vi "close.vi"(8 "error in (no error)":errorcluster, 11 "K2602 in":refnum<class "K2602.lvclass">) -> (0 "error out":errorcluster)   [LabVIEW 2009, in "Hardware.lvlib" / "Channels.lvlib" / "K2602.lvclass"]
doc: "Closes the analog output device."
uses:
  K2602.lvclass
  K2602.lvclass/K2602.ctl
  <instrlib>/Keithley 2600 Series/Keithley 2600 Series.lvlib
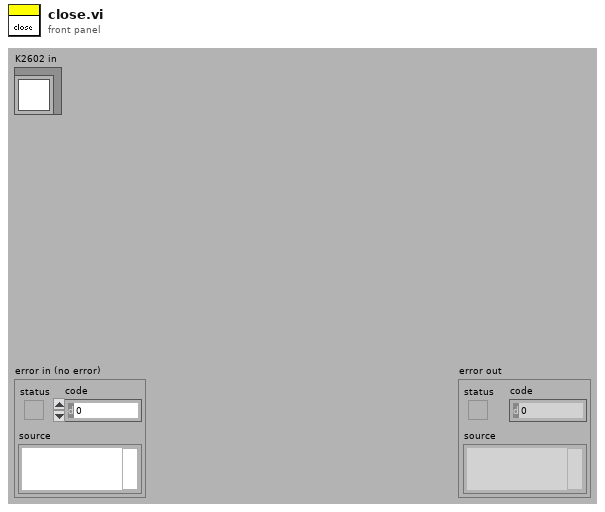
[diagram p1: front panel]
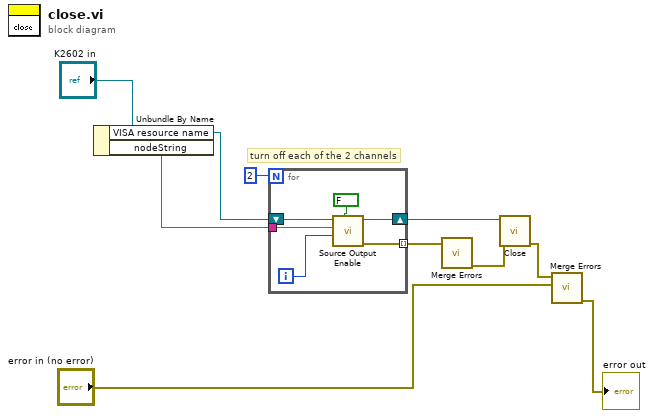
[diagram p0: block diagram]
diagram:
  # "turn off each of the 2 channels"
  n1 = Unbundle By Name("K2602 in") -> ("VISA resource name"=w8:refnum<visa-resource-name>, "nodeString"=w7:string)
  n2 = for {
    N: 2 -> [_]
    tunnel: w7 -> [w13]
    shift-right: [w16] -> w10
    shift-left: w8 -> [w14]
    tunnel: [w11] -> w4 mode=indexing
    i -> [w12]
    n3 = call <instrlib>:"Source Output Enable.vi"("Output (Off)"=FALSE, "Channel (Channel A)"=w12, "Node In"=w13, "VISA resource name"=w14) -> ("error out"=w11:errorcluster, "VISA resource name out"=w16:refnum<visa-resource-name>)  [unwired: 1 in, 5 out]
  }
  n4 = call <vilib>:"Merge Errors.vi"("error array in"=w4) -> ("error out"=w5:errorcluster)  [unwired: 6 in]
  n5 = call <instrlib>:"Close.vi"("error in (no error)"=w5, "VISA resource name"=w10) -> ("error out"=w3:errorcluster)  [unwired: 9 out]
  n6 = call <vilib>:"Merge Errors.vi"("error in 2 (no error)"="error in (no error)", "error in 1 (no error)"=w3) -> ("error out"=→"error out":errorcluster)  [unwired: 5 in]
